vi "Set Sin Wava source (SubVI).vi"(9 "Hz":dbl, 10 "A":dbl, 11 "VISA引用句柄输入":refnum<visa-resource-name>) -> ()   [LabVIEW 2019, in "SubVI.lvlib"]
uses:
  SubVI.lvlib
  lib/Keithley 622x/Configure/6221 Wave/Low Level/Typedefs/KE6221 -- Wave Type.ctl
  lib/Keithley 622x/Keithley 622x.lvlib
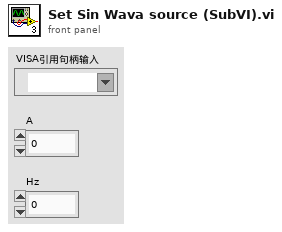
[diagram p1: front panel]
types:
  T1 = typedef "Keithley 622x.lvlib/KE6221 -- Wave Type.ctl" = enum16{"Sinusoid", "Square", "Ramp", "Arbitrary 0", "Arbitrary 1", "Arbitrary 2", "Arbitrary 3", "Arbitrary 4"}
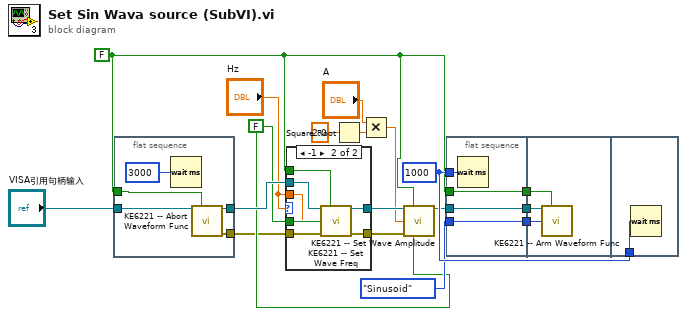
[diagram p0: block diagram]
diagram:
  w15 = u32 1000 ("milliseconds to wait")
  w6 = FALSE ("Read Back Set Value? (T)")
  w11 = FALSE ("Check For SCPI Errors? (T)")
  n1 = flat-sequence {
    tunnel: w11 -> [w23]
    tunnel: [w22] -> w8
    tunnel: "VISA引用句柄输入" -> [w21]
    tunnel: [w20] -> w1
    frame #0 {
      n2 = Wait (ms)(milliseconds to wait=u32 3000 ("等待时间（毫秒）")) -> ()  [unwired: 1 out]
      n3 = call "KE6221 -- Abort Waveform Func.vi"("Resource In"=w21, "Check For SCPI Errors? (T)"=w23) -> ("Resource Out (dupl)"=w22:refnum<visa-resource-name>, "error out"=w20:errorcluster)  [unwired: 12 in]
    }
  }
  n4 = case shown="-1" "Hz" {
    tunnel: w11 -> [_ w32]
    tunnel: w8 -> [w25 w31]
    tunnel: w6 -> [_ w30]
    tunnel: [w24 w29] -> w5
    tunnel: "Hz" -> [_ w28]
    tunnel: [w25 w27] -> w4
    tunnel: w1 -> [w24 w26]
    frame 0, Default {
    }
    frame -1 {
      n5 = call "KE6221 -- Set Wave Freq.vi"("Resource In"=w31, "Check For SCPI Errors? (T)"=w32, "Wave Frequency In (Hz)"=w28, "error in (no error)"=w26, "Read Back Set Value? (T)"=w30) -> ("Resource Out (dupl)"=w27:refnum<visa-resource-name>, "error out"=w29:errorcluster)  [unwired: 8 in, 1 out]
    }
  }
  n6 = Square Root(x=2.0) -> (sqrt(x)=w13:dbl)
  n7 = Multiply(x="A", y=w13) -> (x*y=w3:dbl)
  n8 = call "KE6221 -- Set Wave Amplitude.vi"("Resource In"=w4, "Check For SCPI Errors? (T)"=w11, "Wave Amplitude In"=w3, "error in (no error)"=w5, "Read Back Set Value? (T)"=w6) -> ("Resource Out (dupl)"=w10:refnum<visa-resource-name>)  [unwired: 8 in, 2 out]
  n9 = flat-sequence {
    tunnel: w11 -> [w34]
    tunnel: w10 -> [w35]
    tunnel: KE6221_--_Wave_Type."Sinusoid" ("Wave Type") -> [w36]
    tunnel: [w36] -> w18
    tunnel: [w35] -> w17
    tunnel: [w34] -> w16
    tunnel: w15 -> [w33]
    tunnel: w18 -> [w39]
    tunnel: w17 -> [w38]
    tunnel: w16 -> [w37]
    tunnel: w15 -> [w40]
    frame #0 {
      n10 = Wait (ms)(milliseconds to wait=w33) -> ()  [unwired: 1 out]
    }
    frame #1 {
      n11 = call "KE6221 -- Arm Waveform Func.vi"("Resource In"=w38, "Check For SCPI Errors? (T)"=w37, "Wave Type"=w39) -> ()  [unwired: 11 in, 2 out]
    }
    frame #2 {
      n12 = Wait (ms)(milliseconds to wait=w40) -> ()  [unwired: 1 out]
    }
  }
